vi "from string.vi"(8 "error in":errorcluster, 9 "data":string, 10 "version":string, 11 "Modbus Slave configuration in":refnum<class "Modbus Module configuration.lvclass">) -> (0 "error out":errorcluster, 3 "Modbus Slave configuration out":refnum<class "Modbus Module configuration.lvclass">)   [LabVIEW 2013, in "Modbus Module configuration.lvclass"]
doc: "Provides an interface for loading a module configuration from a file or other serialized data source. It is recommended that all children of this class store data in two sets--data required for its own initialization, and any data required for parent initialization--and that each implementation uses the <b>Call Parent Method</b> primitive to de-serialize parent information. As a result, it is expected that every module configuration class calls <b>component configuration.lvclass:From String.vi</b>.Platypus Framework 1.0.1.65\nNI Systems Engineering - National Instruments"
uses:
  Modbus Module configuration.lvclass
  module channel/Modbus Module Channel.lvclass
  modbus class.ctl
  <vilib>/NI/Tag Bus Module Framework/module configuration/TBM module configuration.lvclass
  Modbus Module configuration.lvclass/Modbus Module configuration.ctl
  <vilib>/NI/Configuration Framework/serializable configuration/NISE_CEF_serializable configuration.lvclass
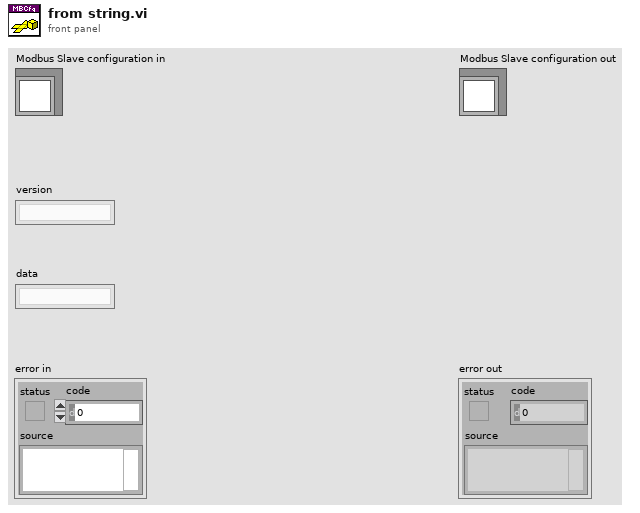
[diagram p1: front panel]
types:
  T1 = typedef "Modbus Module configuration.lvclass/modbus class.ctl" = enum16{"TCP master", "TCP slave", "serial master", "serial slave"}
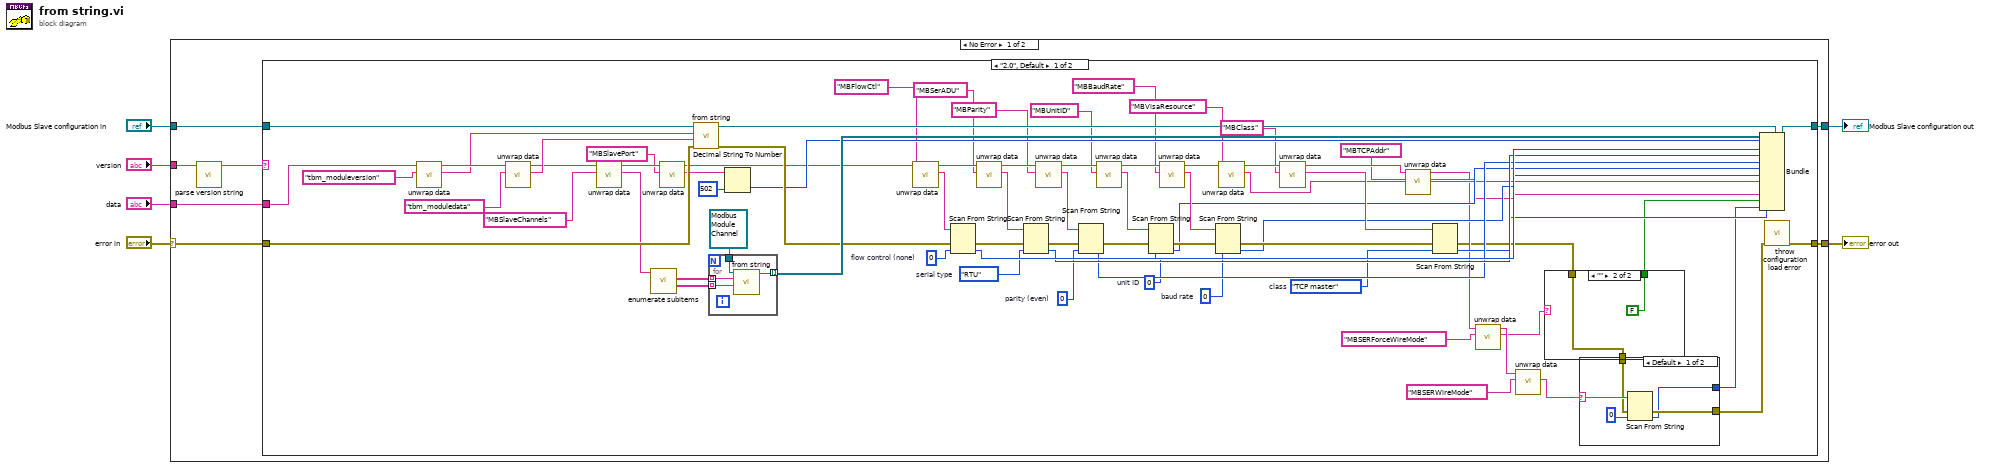
[diagram p0: block diagram]
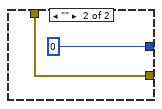
[diagram p2: hidden frame]
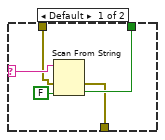
[diagram p3: hidden frame]
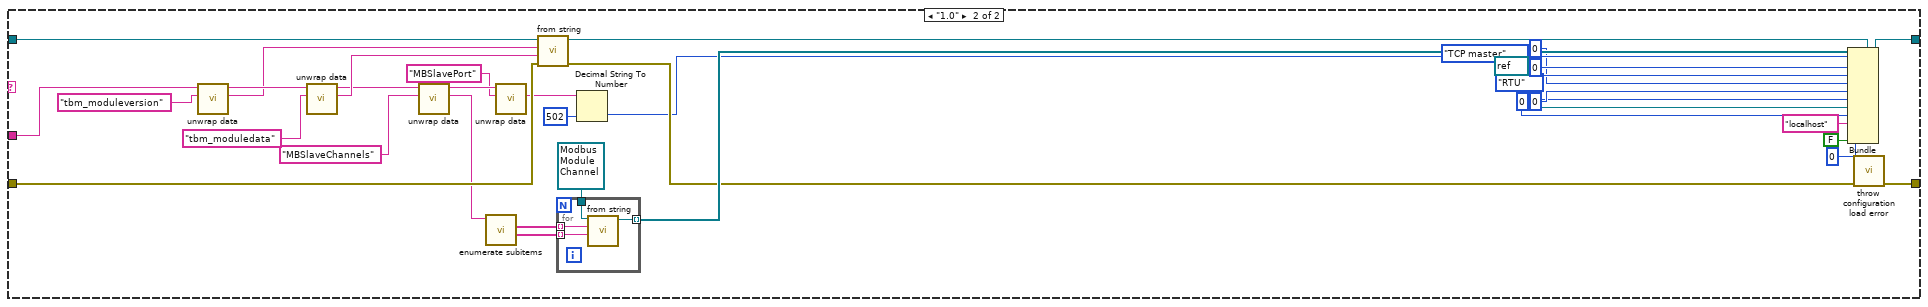
[diagram p4: hidden frame]
diagram:
  n1 = case shown="No Error" "error in" {
    selector: "error in" -> [w7 w147]
    tunnel: "data" -> [w13 _]
    tunnel: "Modbus Slave configuration in" -> [w12 w146]
    tunnel: [w11 w146] -> w5
    tunnel: [w10 w147] -> w4
    tunnel: "version" -> [w9 _]
    frame No Error {
      n2 = call <vilib>:"parse version string.vi"("full version"=w9) -> ("major.minor version"=w8:string)  [unwired: 7 in, 3 out]
      n3 = case shown="\"2.0\", Default" w8 {
        tunnel: w13 -> [w85 w137]
        tunnel: w7 -> [w84 w136]
        tunnel: w12 -> [w89 w141]
        tunnel: [w79 w131] -> w11
        tunnel: [w87 w139] -> w10
        frame "2.0", Default {
          w28 = u32 0  # baud rate
          w29 = modbus_class."TCP master"  # class
          w30 = enum16{"RTU", "ASCII"}."RTU"  # serial type
          w31 = u16 0  # parity (even)
          w32 = u8 0  # unit ID
          w40 = u16 0  # flow control (none)
          n4 = call <vilib>:"unwrap data.vi"("identifier"="tbm_moduleversion" ("additional identifier"), "data to unwrap"=w85) -> ("unwrapped data"=w80:string, "remaining string"=w86:string)  [unwired: 8 in]
          n5 = call <vilib>:"unwrap data.vi"("identifier"="tbm_moduledata" ("additional identifier"), "data to unwrap"=w86) -> ("unwrapped data"=w82:string, "remaining string"=w78:string)  [unwired: 8 in]
          n6 = call <vilib>:"unwrap data.vi"("identifier"="MBSlaveChannels" ("additional identifier"), "data to unwrap"=w78) -> ("unwrapped data"=w76:string, "remaining string"=w71:string)  [unwired: 8 in]
          n7 = call <vilib>:"enumerate subitems.vi"("data to enumerate"=w76) -> ("associated data"=w74:string[], "discovered subitems"=w75:string[])  [unwired: 8 in, 1 out]
          n8 = call <vilib>:"unwrap data.vi"("identifier"="MBSlavePort" ("additional identifier"), "data to unwrap"=w71) -> ("unwrapped data"=w69:string, "remaining string"=w59:string)  [unwired: 8 in]
          n9 = call-parent "from string.vi"("error in"=w84, "data"=w82, "version"=w80, "module configuration in"=w89) -> ("error out"=w72:errorcluster, "module configuration out"=w88:refnum<class "Modbus Module configuration.lvclass">)  [unwired: 6 in]
          n10 = for {
            tunnel: w75 -> [w107] mode=indexing
            tunnel: w74 -> [w106] mode=indexing
            tunnel: [w105] -> w73 mode=indexing
            tunnel: refnum<class "Modbus Module Channel.lvclass"> refnum ("Modbus Module Channel.lvclass") -> [w104]
            n11 = call-dynamic "from string.vi"("channel data"=w106, "identifier"=w107, "channel in"=w104) -> ("channel out"=w105:refnum<class "Modbus Module Channel.lvclass">)  [unwired: 7 in, 1 out]
          }
          n12 = Decimal String To Number(string=w69, default (0L)=u16 502 ("default (0 I32)")) -> (number=w67:u16)  [unwired: 1 in, 1 out]
          n13 = call <vilib>:"unwrap data.vi"("identifier"="MBFlowCtl", "data to unwrap"=w59) -> ("unwrapped data"=w47:string, "remaining string"=w60:string)  [unwired: 8 in]
          n14 = Scan From String(input string=w47, error in=w72, default 1=w40) -> (error out=w50:errorcluster, output 1=w39:u16)  [unwired: 2 in, 2 out]
          n15 = call <vilib>:"unwrap data.vi"("identifier"="MBSerADU", "data to unwrap"=w60) -> ("unwrapped data"=w48:string, "remaining string"=w61:string)  [unwired: 8 in]
          n16 = Scan From String(input string=w48, error in=w50, default 1=w30) -> (error out=w49:errorcluster, output 1=w38:enum16{"RTU", "ASCII"})  [unwired: 2 in, 2 out]
          n17 = call <vilib>:"unwrap data.vi"("identifier"="MBParity", "data to unwrap"=w61) -> ("unwrapped data"=w46:string, "remaining string"=w62:string)  [unwired: 8 in]
          n18 = Scan From String(input string=w46, error in=w49, default 1=w31) -> (error out=w51:errorcluster, output 1=w37:u16)  [unwired: 2 in, 2 out]
          n19 = call <vilib>:"unwrap data.vi"("identifier"="MBUnitID", "data to unwrap"=w62) -> ("unwrapped data"=w44:string, "remaining string"=w63:string)  [unwired: 8 in]
          n20 = Scan From String(input string=w44, error in=w51, default 1=w32) -> (error out=w45:errorcluster, output 1=w36:u8)  [unwired: 2 in, 2 out]
          n21 = call <vilib>:"unwrap data.vi"("identifier"="MBBaudRate", "data to unwrap"=w63) -> ("unwrapped data"=w42:string, "remaining string"=w64:string)  [unwired: 8 in]
          n22 = Scan From String(input string=w42, error in=w45, default 1=w28) -> (error out=w43:errorcluster, output 1=w35:u32)  [unwired: 2 in, 2 out]
          n23 = call <vilib>:"unwrap data.vi"("identifier"="MBVisaResource", "data to unwrap"=w64) -> ("unwrapped data"=w33:string, "remaining string"=w65:string)  [unwired: 8 in]
          n24 = call <vilib>:"unwrap data.vi"("identifier"="MBClass", "data to unwrap"=w65) -> ("unwrapped data"=w41:string, "remaining string"=w27:string)  [unwired: 8 in]
          n25 = call <vilib>:"unwrap data.vi"("identifier"="MBTCPAddr", "data to unwrap"=w27) -> ("unwrapped data"=w25:string, "remaining string"=w24:string)  [unwired: 8 in]
          n26 = Scan From String(input string=w41, error in=w43, default 1=w29) -> (error out=w16:errorcluster, output 1=w34:T1)  [unwired: 2 in, 2 out]
          n27 = call <vilib>:"unwrap data.vi"("identifier"="MBSERForceWireMode", "data to unwrap"=w24) -> ("unwrapped data"=w20:string, "remaining string"=w23:string)  [unwired: 8 in]
          n28 = call <vilib>:"unwrap data.vi"("identifier"="MBSERWireMode", "data to unwrap"=w23) -> ("unwrapped data"=w19:string)  [unwired: 8 in, 1 out]
          n29 = case shown="\"\"" w20 {
            selector: w20 -> [w101 _]
            tunnel: [w99 FALSE] -> w17
            tunnel: w16 -> [w98 w102]
            tunnel: [w97 w102] -> w15
            frame Default {
              n30 = Scan From String(input string=w101, error in=w98, default 1=FALSE) -> (error out=w97:errorcluster, output 1=w99:bool)  [unwired: 2 in, 2 out]
            }
            frame "" {
            }
          }
          n31 = case shown="Default" w19 {
            selector: w19 -> [w94 _]
            tunnel: [w90 i16 0 ("Wire Mode")] -> w18
            tunnel: w15 -> [w92 w95]
            tunnel: [w91 w95] -> w14
            frame Default {
              n32 = Scan From String(input string=w94, error in=w92, default 1=i16 0 ("Wire Mode")) -> (error out=w91:errorcluster, output 1=w90:i16)  [unwired: 2 in, 2 out]
            }
            frame "" {
            }
          }
          n33 = Bundle(cluster=w88, w73, w67, w39, w38, w37, w36, w35, w33, w34, w25, w17, w18) -> (w79:refnum<class "Modbus Module configuration.lvclass">)
          n34 = call <vilib>:"throw configuration load error.vi"("error in"=w14) -> ("error out"=w87:errorcluster)  [unwired: 10 in]
        }
        frame "1.0" {
          n35 = call <vilib>:"unwrap data.vi"("identifier"="tbm_moduleversion" ("additional identifier"), "data to unwrap"=w137) -> ("unwrapped data"=w132:string, "remaining string"=w138:string)  [unwired: 8 in]
          n36 = call <vilib>:"unwrap data.vi"("identifier"="tbm_moduledata" ("additional identifier"), "data to unwrap"=w138) -> ("unwrapped data"=w134:string, "remaining string"=w130:string)  [unwired: 8 in]
          n37 = call <vilib>:"unwrap data.vi"("identifier"="MBSlaveChannels" ("additional identifier"), "data to unwrap"=w130) -> ("unwrapped data"=w128:string, "remaining string"=w123:string)  [unwired: 8 in]
          n38 = call <vilib>:"enumerate subitems.vi"("data to enumerate"=w128) -> ("associated data"=w126:string[], "discovered subitems"=w127:string[])  [unwired: 8 in, 1 out]
          n39 = call <vilib>:"unwrap data.vi"("identifier"="MBSlavePort" ("additional identifier"), "data to unwrap"=w123) -> ("unwrapped data"=w121:string)  [unwired: 8 in, 1 out]
          n40 = call-parent "from string.vi"("error in"=w136, "data"=w134, "version"=w132, "module configuration in"=w141) -> ("error out"=w124:errorcluster, "module configuration out"=w140:refnum<class "Modbus Module configuration.lvclass">)  [unwired: 6 in]
          n41 = for {
            tunnel: w127 -> [w145] mode=indexing
            tunnel: w126 -> [w144] mode=indexing
            tunnel: [w143] -> w125 mode=indexing
            tunnel: refnum<class "Modbus Module Channel.lvclass"> refnum ("Modbus Module Channel.lvclass") -> [w142]
            n42 = call-dynamic "from string.vi"("channel data"=w144, "identifier"=w145, "channel in"=w142) -> ("channel out"=w143:refnum<class "Modbus Module Channel.lvclass">)  [unwired: 7 in, 1 out]
          }
          n43 = Decimal String To Number(string=w121, default (0L)=u16 502 ("default (0 I32)")) -> (number=w119:u16)  [unwired: 1 in, 1 out]
          n44 = Bundle(cluster=w140, w125, w119, u16 0 ("flow control (none)"), enum16{"RTU", "ASCII"}."RTU" ("serial type"), u16 0 ("parity (even)"), u8 0 ("unit ID"), u32 0 ("baud rate"), refnum<visa-resource-name> refnum ("VISA resource name"), modbus_class."TCP master" ("class"), "localhost" ("IP address"), FALSE ("force wire mode"), i16 0 ("Wire Mode")) -> (w131:refnum<class "Modbus Module configuration.lvclass">)
          n45 = call <vilib>:"throw configuration load error.vi"("error in"=w124) -> ("error out"=w139:errorcluster)  [unwired: 10 in]
        }
      }
    }
    frame Error {
    }
  }
  "error out" <- w4
  "Modbus Slave configuration out" <- w5
